vi "GetTrendList.vi"() -> (2 "Y列表":string[](array[string]), 3 "X列表":string[](array[string]))   [LabVIEW 2018, in "DataDisplay.lvlib" / "TrendPlot.lvclass"]
uses:
  TrendPlot.lvclass
  SubVI/DD_Parameter.vi
  DataDisplay.lvlib
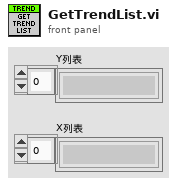
[diagram p1: front panel]
types:
  T1 = typedef "DataDisplay.lvlib/DD_ChannelInfo.ctl" = cluster{"名称":string, "单位":string, "数据类型":enum16{"Real", "Int"}, "趋势线":enum16{"N/A", "X", "Y"}}
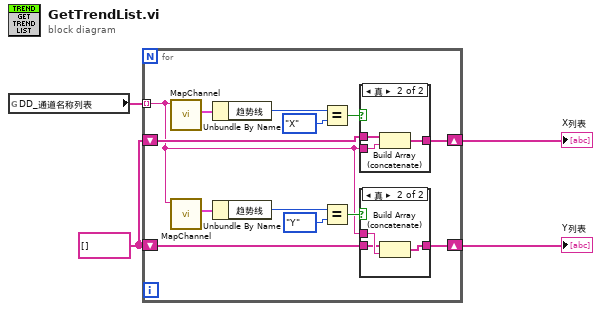
[diagram p0: block diagram]
diagram:
  w4 = string[] []
  n1 = global read "DD_Parameter.vi" "DD_通道名称列表"() -> (w1:string[])
  n2 = for {
    tunnel: w1 -> [w5] mode=indexing
    shift-right: [w12] -> w2
    shift-left: w4 -> [w13]
    shift-right: [w6] -> w3
    shift-left: w4 -> [w7]
    n3 = call "MapChannel.vi"("通道名称"=w5) -> ("通道信息"=w8:T1)  [unwired: 9 in, 1 out]
    n4 = call "MapChannel.vi"("通道名称"=w5) -> ("通道信息"=w17:T1)  [unwired: 9 in, 1 out]
    n5 = Unbundle By Name(w8) -> ("趋势线"=w9:enum16{"N/A", "X", "Y"})
    n6 = Unbundle By Name(w17) -> ("趋势线"=w16:enum16{"N/A", "X", "Y"})
    n7 = Equal?(x=w9, y=enum16{"N/A", "X", "Y"}."X") -> (x = y?=w11:bool)
    n8 = Equal?(x=w16, y=enum16{"N/A", "X", "Y"}."Y") -> (x = y?=w14:bool)
    n9 = case shown="真" w11 {
      tunnel: w5 -> [_ w21]
      tunnel: w7 -> [w18 w20]
      tunnel: [w18 w19] -> w6
      frame False {
      }
      frame True {
        n10 = Build Array (concatenate)(w20, w21) -> (w19:string[])
      }
    }
    n11 = case shown="真" w14 {
      tunnel: w5 -> [_ w25]
      tunnel: w13 -> [w22 w24]
      tunnel: [w22 w23] -> w12
      frame False {
      }
      frame True {
        n12 = Build Array (concatenate)(w24, w25) -> (w23:string[])
      }
    }
  }
  "X列表" <- w3
  "Y列表" <- w2
